vi "RMSE_Rotation.vi"(7 "Values":T3, 8 "mask":i32[][](array[numeric]), 9 "rev/s":dbl, 10 "Coord Grid":cdb[][](array[numeric]), 11 "V m/s":cdb[][][](array[numeric])) -> ()   [LabVIEW 2022 SP3]
uses:
  <vilib>/Utility/miscctls.llb/LVPointDoubleTypeDef.ctl
  <vilib>/Analysis/5stat.llb/RMS (DBL).vi
  <vilib>/Analysis/2dsp.llb/Decimate (single shot, DBL).vi
  <vilib>/Utility/file.llb/Write Delimited Spreadsheet (DBL).vi
  <vilib>/Analysis/NI_AALPro.lvlib
  <vilib>/Analysis/NI_AALBase.lvlib
panel:
  in  "Angles":i32[](array[numeric])=[0, 45]
  in  "multi angles":bool
  in  "Xtra Data Shift":T1
  out "ideal V cm/s":dbl[][](graph)
  in  "Tab Control":T2(tab)
  out "A1 Mean phase":dbl[][](graph)
  out "A1 Mean Vx":dbl[][](graph)
  out "AMean Vy":dbl[][](graph)
  out "A1 Mean V":dbl[][](graph)
  out "A2 Mean V":dbl[][](graph)
  out "A2 Mean Vy":dbl[][](graph)
  out "A2 Mean Vx":dbl[][](graph)
  out "A2 Mean phase":dbl[][](graph)
  out "Angles":i32[](array[numeric])
  out "ideal V_y cm/s 2":dbl[][](graph)
  out "ideal V_y cm/s":dbl[][](graph)
  out "ideal V_xcm/s":dbl[][](graph)
  out "RMSE V cm/s":dbl[][](graph)
  out "RMSE Phase (degrees)":dbl[][](graph)
  out "RMSE V_x cm/s":dbl[][](graph)
  out "RMSE  V_y cm/s":dbl[][](graph)
  out "Mean V cm/s":dbl[][](graph)
  out "Mean Phase":dbl[][](graph)
  out "Mean V _x cm/s":dbl[][](graph)
  out "Mean V y cm/s":dbl[][](graph)
  out "SD V cm/s":dbl[][](graph)
  out "SD Phase":dbl[][](graph)
  out "SD V_x cm/s":dbl[][](graph)
  out "SD V_y cm/s":dbl[][](graph)
  in  "Save":bool
  in  "Clockwise Rotate angle":i32
  in  "Pad Pts":i32=1
  out "Average RMSE Phase":dbl
  out "Average RMSE":dbl
  out "Max V":dbl
  in  "Scale?":bool
  in  "Operation":u16(ring) items=["Median", "Mean"]
  in  "median size":dbl=3.0
  # "9 and 5 tested"
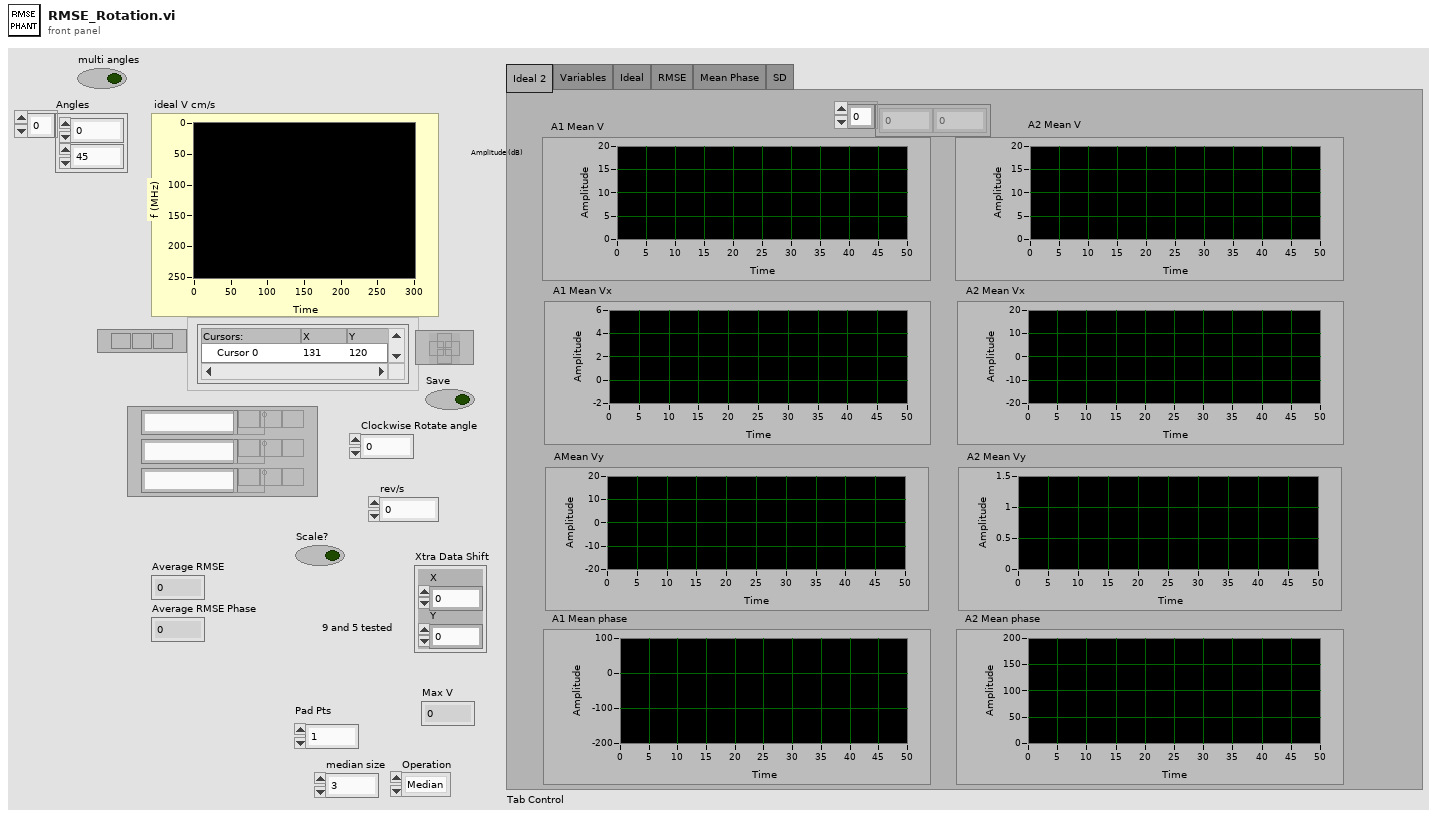
[diagram p1: front panel]
types:
  T1 = typedef "LVPointDoubleTypeDef.ctl" = cluster{"X":dbl, "Y":dbl}
  T2 = enum32{"Ideal 2", "Variables", "Ideal", "RMSE", "Mean Phase", "SD"}
  T3 = cluster{"xdim":dbl, "ydim":dbl, "zdim":dbl, "skip":dbl, "ensembleC":dbl, "ensembleVar\n":dbl, "#tx":dbl, "#Rx":dbl, "deltaX":dbl, "deltaY":dbl, "x start":dbl, "ystart":dbl}
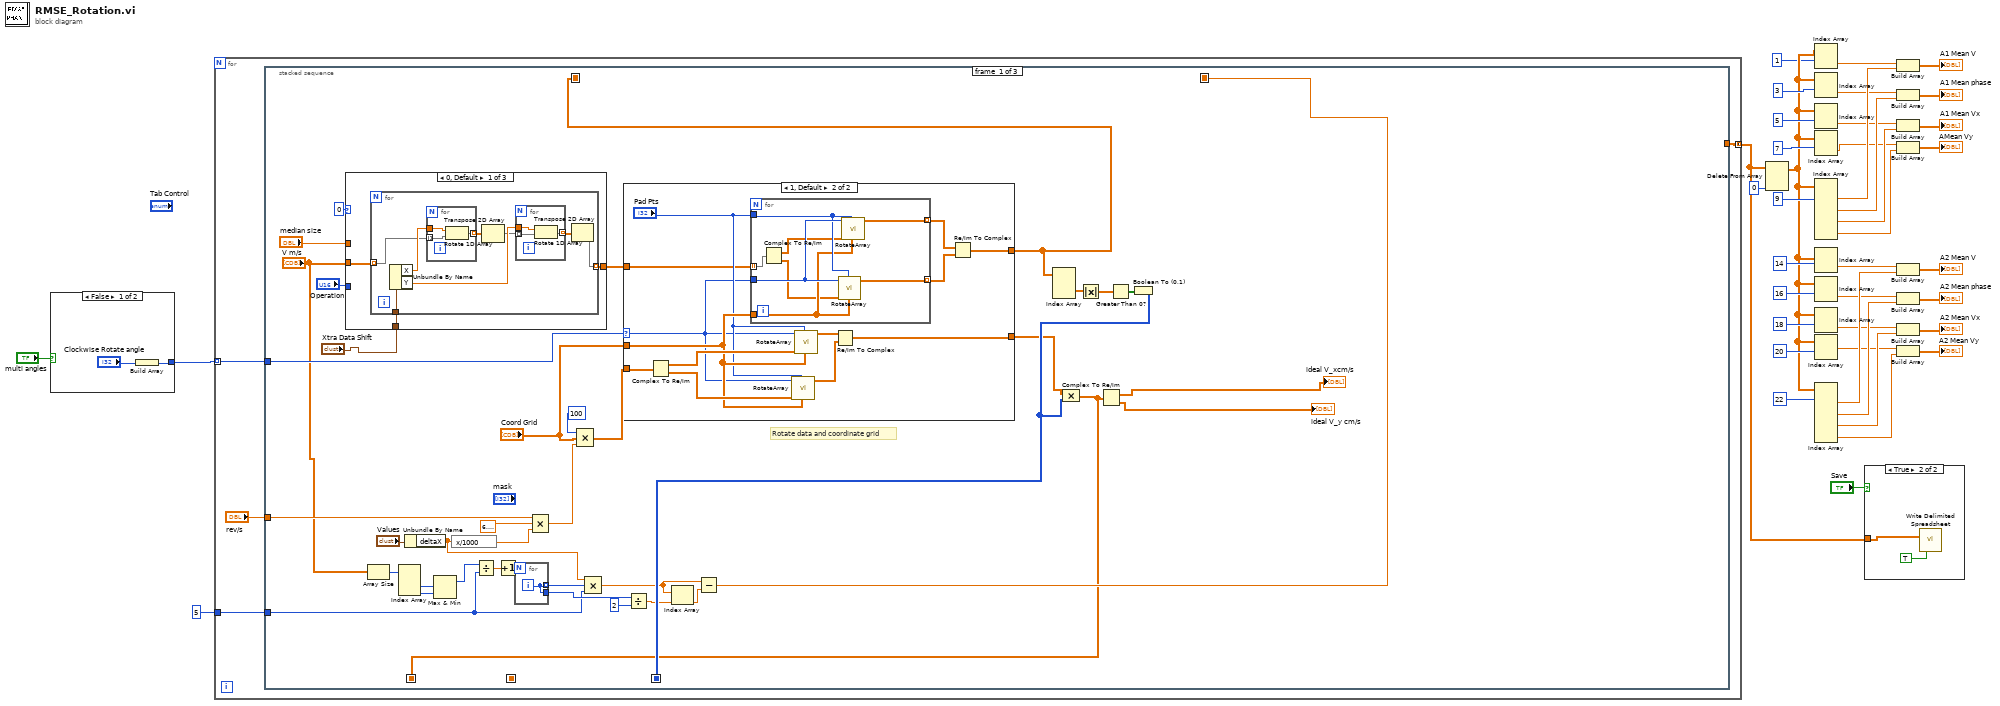
[diagram p0: block diagram]
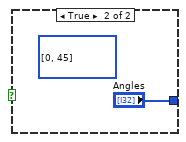
[diagram p2: hidden frame]
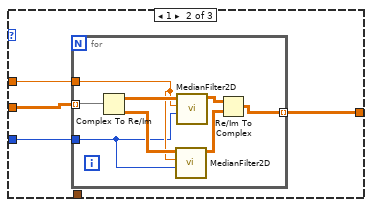
[diagram p4: hidden frame]
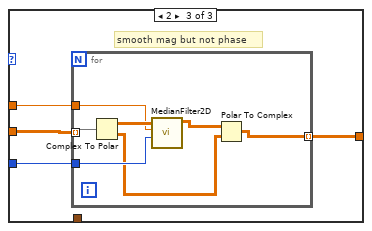
[diagram p5: hidden frame]
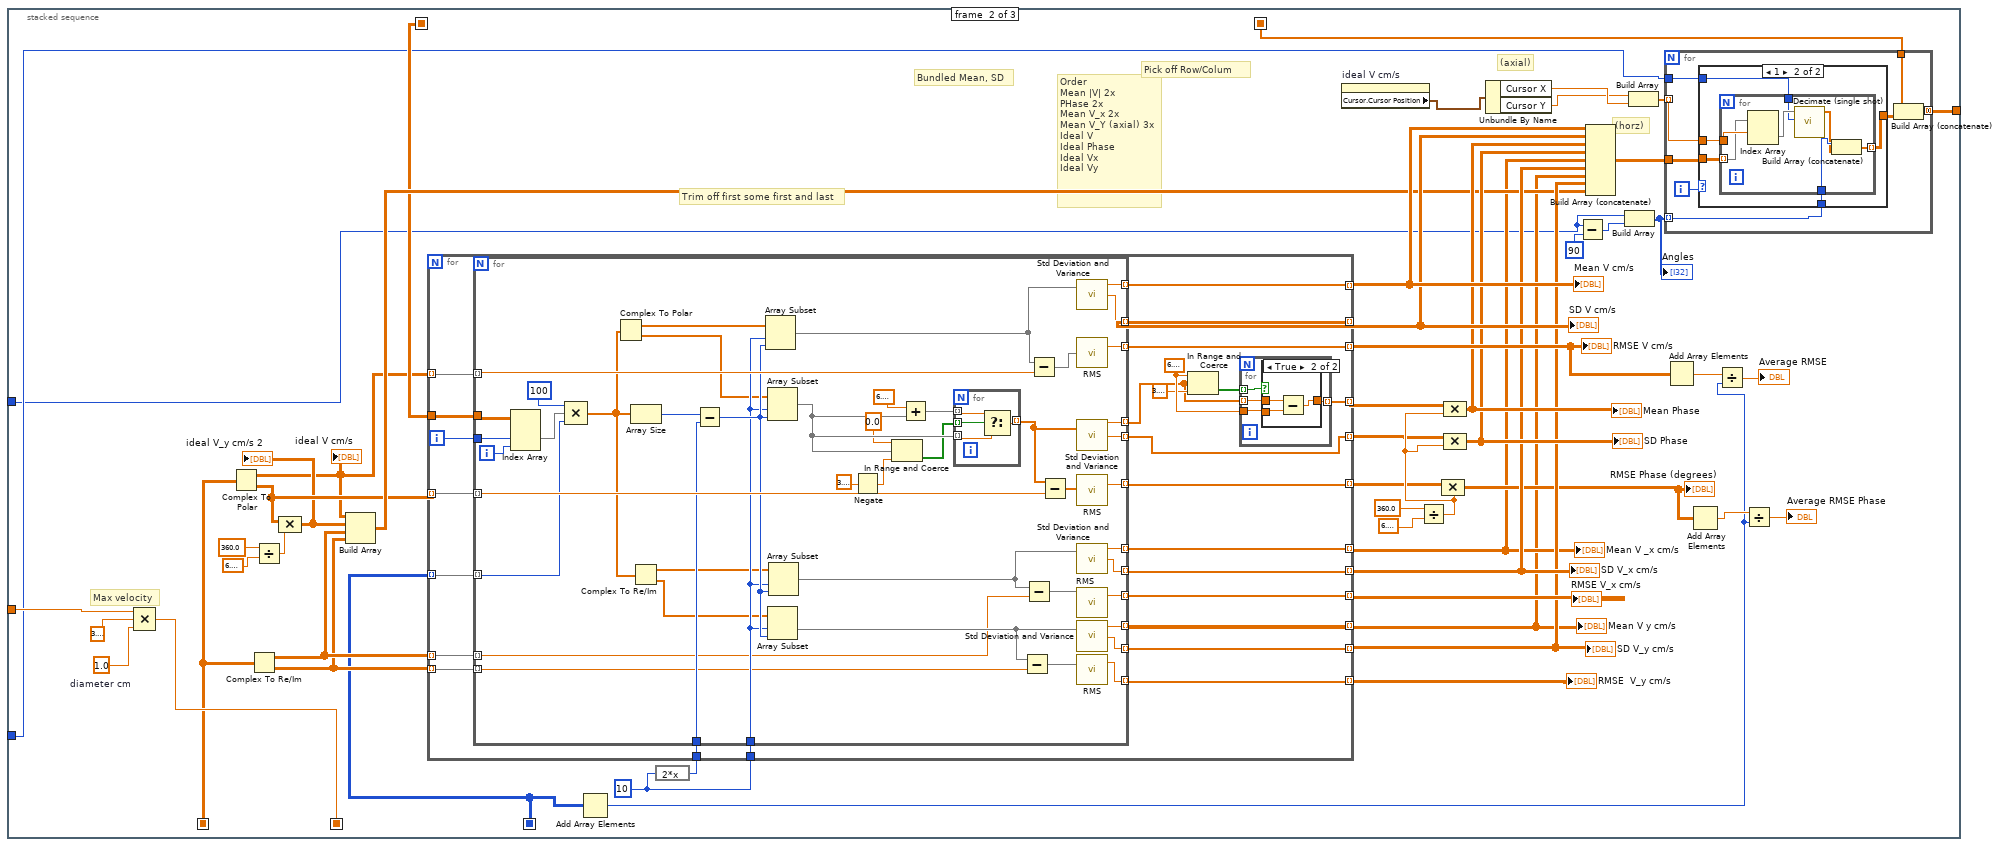
[diagram p6: hidden frame]
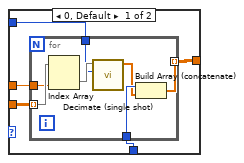
[diagram p7: hidden frame]
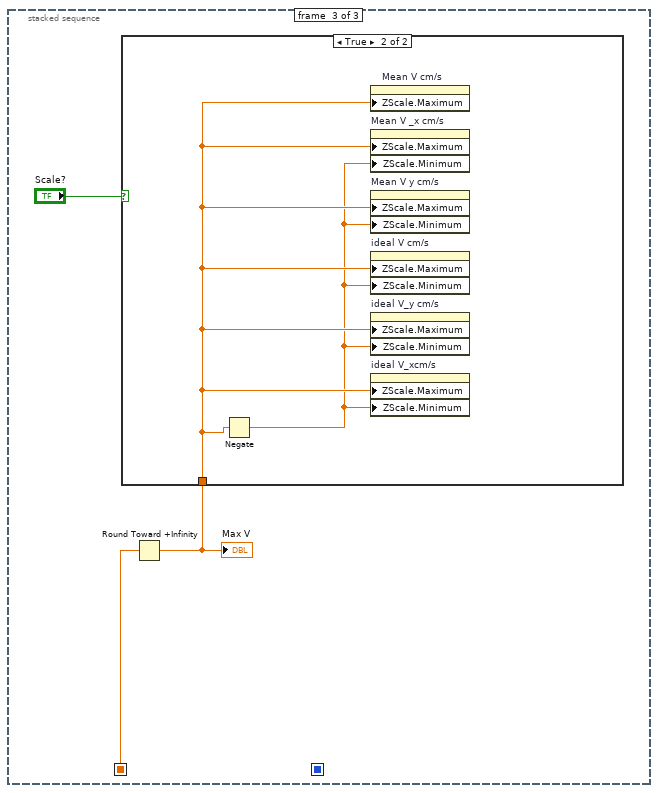
[diagram p9: hidden frame]
diagram:
  n1 = case shown="False" "multi angles" {
    tunnel: [w42 "Angles"] -> w7
    frame False {
      n2 = Build Array("Clockwise Rotate angle") -> (w42:i32[])
    }
    frame True {
      (unwired) i32[] [0, 45]
    }
  }
  n3 = for {
    tunnel: w7 -> [w47] mode=indexing
    tunnel: [w46] -> w6 mode=concatenating
    tunnel: 5 ("y") -> [w45]
    n4 = stacked-sequence {
      seq-local: [_ w170 _] -> [_ _ w321]
      seq-local: [w50 _ _] -> [_ w161 _]
      seq-local: [w73 _ _] -> [_ w168 _]
      seq-local: [w49 _ _] -> [_ w162 _]
      seq-local: [w61 _ _] -> [_ w160 _]
      tunnel: [_ w165 _] -> w46
      tunnel: "rev/s" -> [w79 w169 _]
      tunnel: w47 -> [w70 w158 _]
      tunnel: w45 -> [w53 w159 _]
      frame #0 {
        # "Rotate data and coordinate grid"
        n5 = case shown="0, Default" 0 {
          tunnel: "V m/s" -> [w114 w132 w144]
          tunnel: "median size" -> [_ w131 w143]
          tunnel: "Operation" -> [_ w130 w142]
          tunnel: [w113 w129 w141] -> w87
          tunnel: "Xtra Data Shift" -> [w112 _ _]
          frame 0, Default {
            n6 = for {
              tunnel: w114 -> [w117] mode=indexing
              tunnel: [w116] -> w113 mode=indexing
              tunnel: w112 -> [w115]
              n7 = Unbundle By Name(w115) -> ("X"=w121:dbl, "Y"=w122:dbl)
              n8 = for {
                tunnel: [w128] -> w118 mode=indexing
                tunnel: w121 -> [w127]
                tunnel: w117 -> [w126] mode=indexing
                n9 = Rotate 1D Array(1:w126, 2:w127) -> (0:w128:cdb[])
              }
              n10 = Transpose 2D Array(2D array=w118) -> (transposed array=w119:cdb[][])
              n11 = for {
                tunnel: w119 -> [w125] mode=indexing
                tunnel: [w124] -> w120 mode=indexing
                tunnel: w122 -> [w123]
                n12 = Rotate 1D Array(1:w125, 2:w123) -> (0:w124:cdb[])
              }
              n13 = Transpose 2D Array(2D array=w120) -> (transposed array=w116:cdb[][])
            }
          }
          frame 1 {
            n14 = for {
              tunnel: w132 -> [w140] mode=indexing
              tunnel: w131 -> [w134]
              tunnel: w130 -> [w133]
              tunnel: [w137] -> w129 mode=indexing
              n15 = Complex To Re/Im(x + iy=w140) -> (x=w139:dbl[][], y=w136:dbl[][])
              n16 = call "MedianFilter2D.vi"("Operation"=w133, "Pts to use"=w134, "Raw In"=w136) -> ("output array"=w135:sgl[][])  [unwired: 8 in]
              n17 = call "MedianFilter2D.vi"("Operation"=w133, "Pts to use"=w134, "Raw In"=w139) -> ("output array"=w138:sgl[][])  [unwired: 8 in]
              n18 = Re/Im To Complex(1:w135, 2:w138) -> (0:w137:csg[][])
            }
          }
          frame 2 {
            # "smooth mag but not phase"
            n19 = for {
              tunnel: w144 -> [w151] mode=indexing
              tunnel: w143 -> [w147]
              tunnel: w142 -> [w146]
              tunnel: [w148] -> w141 mode=indexing
              n20 = Complex To Polar(r * e^(i*theta)=w151) -> (r=w150:dbl[][], theta=w145:dbl[][])
              n21 = call "MedianFilter2D.vi"("Operation"=w146, "Pts to use"=w147, "Raw In"=w150) -> ("output array"=w149:sgl[][])  [unwired: 8 in]
              n22 = Polar To Complex(1:w145, 2:w149) -> (0:w148:cdb[][])
            }
          }
        }
        n23 = Array Size(array="V m/s") -> (size(s)=w59:i32[])
        n24 = Index Array(array=w59) -> (element #2=w56:i32, element #3=w55:i32)  [unwired: 3 in, 1 out]
        n25 = Unbundle By Name("Values") -> ("deltaX"=w67:dbl)
        n26 = Max & Min(x=w56, y=w55) -> (max(x,y)=w54:i32)  [unwired: 1 out]
        n27 = expression code="x/1000"(w67) -> (w80:dbl)
        n28 = Divide(x=w54, y=w53) -> (x/y=w58:dbl)
        n29 = Increment(x=w58) -> (x+1=w57:dbl)
        n30 = for {
          N: w57 -> [_]
          tunnel: [w88] -> w68 mode=indexing
          tunnel: [w88] -> w66
          i -> [w88]
        }
        n31 = Compound Arithmetic op=MULTIPLY(w79, 6.283185307179586, w80) -> (w77:dbl)
        n32 = Compound Arithmetic op=MULTIPLY(100, "Coord Grid", w77) -> (w69:cdb[][])
        n33 = Compound Arithmetic op=MULTIPLY(w67, w68, w53) -> (w63:dbl[])
        n34 = case shown="1, Default" w70 {
          selector: w70 -> [_ w93]
          tunnel: w87 -> [w90 w91]
          tunnel: [w90 w101] -> w50
          tunnel: "Coord Grid" -> [_ w95]
          tunnel: [w89 w96] -> w51
          tunnel: w69 -> [w89 w92]
          frame 0 {
          }
          frame 1, Default {
            n35 = Complex To Re/Im(x + iy=w92) -> (x=w100:dbl[][], y=w99:dbl[][])
            n36 = for {
              tunnel: [w111] -> w103 mode=indexing
              tunnel: [w110] -> w102 mode=indexing
              tunnel: w93 -> [w109]
              tunnel: w95 -> [w107]
              tunnel: "Pad Pts" -> [w108]
              tunnel: w91 -> [w104] mode=indexing
              n37 = Complex To Re/Im(x + iy=w104) -> (x=w106:dbl[][], y=w105:dbl[][])
              n38 = call "RotateArray.vi"("Vel grid Ideal"=w107, "Pad Pts"=w108, "Peak V in"=w105, "Angle"=w109) -> ("Peak V out"=w110:dbl[][])  [unwired: 6 in, 1 out]
              n39 = call "RotateArray.vi"("Vel grid Ideal"=w107, "Pad Pts"=w108, "Peak V in"=w106, "Angle"=w109) -> ("Peak V out"=w111:dbl[][])  [unwired: 6 in, 1 out]
            }
            n40 = call "RotateArray.vi"("Vel grid Ideal"=w95, "Pad Pts"="Pad Pts", "Peak V in"=w99, "Angle"=w93) -> ("Peak V out"=w97:dbl[][])  [unwired: 6 in, 1 out]
            n41 = call "RotateArray.vi"("Vel grid Ideal"=w95, "Pad Pts"="Pad Pts", "Peak V in"=w100, "Angle"=w93) -> ("Peak V out"=w98:dbl[][])  [unwired: 6 in, 1 out]
            n42 = Re/Im To Complex(1:w97, 2:w98) -> (0:w96:cdb[][])
            n43 = Re/Im To Complex(1:w102, 2:w103) -> (0:w101:cdb[][][])
          }
        }
        n44 = Divide(x=w66, y=2) -> (x/y=w64:dbl)
        n45 = Index Array(array=w63, index=w64) -> (element=w62:dbl)
        n46 = Subtract(x=w63, y=w62) -> (x-y=w61:dbl[])
        n47 = Index Array(array=w50) -> (element=w76:cdb[][])  [unwired: 3 in]
        n48 = Absolute Value(x=w76) -> (abs(x)=w75:dbl[][])
        n49 = Greater Than 0?(x=w75) -> (x > 0?=w74:bool[][])
        n50 = Boolean To (0,1)(Boolean=w74) -> (0, 1=w73:i16[][])
        n51 = Compound Arithmetic op=MULTIPLY(w51, w73) -> (w49:cdb[][])
        n52 = Complex To Re/Im(x + iy=w49) -> (x=→"ideal V_xcm/s":dbl[][], y=→"ideal V_y cm/s":dbl[][])
      }
      frame #1 {
        w171 = 1.0  # diameter cm
        w201 = 10
        # "(horz)"
        # "(axial)"
        # "Pick off Row/Colum"
        # "Order\nMean |V| 2x\nPHase 2x\nMean V_x 2x\nMean V_Y (axial) 3x\nIdeal V\nIdeal Phase\nIdeal Vx\nIdeal Vy"
        # "Bundled Mean, SD"
        # "Max velocity"
        # "Trim off first some first and last"
        n53 = Compound Arithmetic op=MULTIPLY(w169, 3.141592653589793, w171) -> (w170:dbl)
        n54 = Complex To Polar(r * e^(i*theta)=w162) -> (r=w152:dbl[][], theta=w154:dbl[][])
        "ideal V cm/s" <- w152
        n55 = Complex To Re/Im(x + iy=w162) -> (x=w177:dbl[][], y=w176:dbl[][])
        n56 = Divide(x=360.0, y=6.283185307179586) -> (x/y=w179:dbl)
        n57 = Compound Arithmetic op=MULTIPLY(w154, w179) -> (w153:dbl[][])
        "ideal V_y cm/s 2" <- w153
        n58 = Build Array(w152, w153, w177, w176) -> (w178:dbl[][][])
        n59 = Add Array Elements(numeric array=w168) -> (sum=w195:i16)
        n60 = expression code="2*x"(w201) -> (w202:i32)
        n61 = for {
          tunnel: [w245] -> w192 mode=indexing
          tunnel: [w260] -> w188 mode=indexing
          tunnel: w152 -> [w259] mode=indexing
          tunnel: w154 -> [w258] mode=indexing
          tunnel: w202 -> [w257]
          tunnel: w201 -> [w256]
          tunnel: [w244] -> w194 mode=indexing
          tunnel: [w255] -> w193 mode=indexing
          tunnel: [w239] -> w173 mode=indexing
          tunnel: [w238] -> w191 mode=indexing
          tunnel: [w254] -> w186 mode=indexing
          tunnel: [w253] -> w175 mode=indexing
          tunnel: [w252] -> w184 mode=indexing
          tunnel: [w251] -> w174 mode=indexing
          tunnel: [w250] -> w185 mode=indexing
          tunnel: [w249] -> w187 mode=indexing
          tunnel: w168 -> [w248] mode=indexing
          tunnel: w177 -> [w247] mode=indexing
          tunnel: w176 -> [w246] mode=indexing
          tunnel: w161 -> [w243]
          i -> [w261]
          w241 = 6.283185307179586
          n62 = for {
            tunnel: w243 -> [w315]
            tunnel: w261 -> [w314]
            tunnel: [w311] -> w245 mode=indexing
            tunnel: [w310] -> w260 mode=indexing
            tunnel: w259 -> [w309] mode=indexing
            tunnel: w258 -> [w308] mode=indexing
            tunnel: w257 -> [w306]
            tunnel: w256 -> [w298]
            tunnel: [w303] -> w244 mode=indexing
            tunnel: [w300] -> w255 mode=indexing
            tunnel: [w302] -> w237 mode=indexing
            tunnel: [w301] -> w238 mode=indexing
            tunnel: [w291] -> w254 mode=indexing
            tunnel: [w290] -> w253 mode=indexing
            tunnel: [w283] -> w252 mode=indexing
            tunnel: [w286] -> w251 mode=indexing
            tunnel: [w285] -> w250 mode=indexing
            tunnel: [w284] -> w249 mode=indexing
            tunnel: w248 -> [w280] mode=indexing
            tunnel: w247 -> [w282] mode=indexing
            tunnel: w246 -> [w281] mode=indexing
            i -> [w313]
            n63 = Index Array(array=w315, index (dim 1)=w314, index (dim 2)=w313) -> (element=w289:cdb[])  [unwired: 1 in]
            n64 = Compound Arithmetic op=MULTIPLY(100, w289, w280) -> (w287:cdb[])
            n65 = Complex To Polar(r * e^(i*theta)=w287) -> (r=w305:dbl[], theta=w271:dbl[])
            n66 = Array Size(array=w287) -> (size(s)=w307:i32)
            n67 = Complex To Re/Im(x + iy=w287) -> (x=w297:dbl[], y=w296:dbl[])
            n68 = Subtract(x=w307, y=w306) -> (x-y=w299:i32)
            n69 = Array Subset(array=w305, index=w298, length=w299) -> (w304:dbl[])
            n70 = Array Subset(array=w271, index=w298, length=w299) -> (w275:dbl[])
            n71 = Array Subset(array=w296, index=w298, length=w299) -> (w293:dbl[])
            n72 = Array Subset(array=w297, index=w298, length=w299) -> (w292:dbl[])
            n73 = Negate(x=3.141592653589793) -> (-x=w276:dbl)
            n74 = In Range and Coerce(upper limit=0.0, x=w275, lower limit=w276) -> (In Range?=w274:bool[])  [unwired: 1 out]
            n75 = Add(x=6.283185307179586, y=w275) -> (x+y=w273:dbl[])
            n76 = for {
              tunnel: w274 -> [w319] mode=indexing
              tunnel: w275 -> [w317] mode=indexing
              tunnel: w273 -> [w318] mode=indexing
              tunnel: [w316] -> w272 mode=indexing
              n77 = Select(t=w318, s=w319, f=w317) -> (s? t:f=w316:dbl)
            }
            n78 = Subtract(x=w293, y=w281) -> (x-y=w294:dbl[])
            n79 = Subtract(x=w292, y=w282) -> (x-y=w295:dbl[])
            n80 = Subtract(x=w304, y=w309) -> (x-y=w279:dbl[])
            n81 = Subtract(x=w272, y=w308) -> (x-y=w312:dbl[])
            n82 = call <vilib>:"Std Deviation and Variance.vi"("X"=w304) -> ("mean"=w303:dbl, "standard deviation"=w300:dbl)  [unwired: 1 in, 1 out]
            n83 = call-poly <vilib>:"RMS.vi"("X"=w279) -> ("rms value"=w311:dbl)  [unwired: 1 out]
            n84 = call <vilib>:"Std Deviation and Variance.vi"("X"=w272) -> ("mean"=w302:dbl, "standard deviation"=w301:dbl)  [unwired: 1 in, 1 out]
            n85 = call-poly <vilib>:"RMS.vi"("X"=w312) -> ("rms value"=w310:dbl)  [unwired: 1 out]
            n86 = call <vilib>:"Std Deviation and Variance.vi"("X"=w292) -> ("mean"=w290:dbl, "standard deviation"=w284:dbl)  [unwired: 1 in, 1 out]
            n87 = call-poly <vilib>:"RMS.vi"("X"=w295) -> ("rms value"=w291:dbl)  [unwired: 1 out]
            n88 = call <vilib>:"Std Deviation and Variance.vi"("X"=w293) -> ("mean"=w286:dbl, "standard deviation"=w285:dbl)  [unwired: 1 in, 1 out]
            n89 = call-poly <vilib>:"RMS.vi"("X"=w294) -> ("rms value"=w283:dbl)  [unwired: 1 out]
          }
          n90 = In Range and Coerce(upper limit=w241, x=w237, lower limit=3.141592653589793) -> (In Range?=w242:bool[])  [unwired: 1 out]
          n91 = for {
            tunnel: w242 -> [w265] mode=indexing
            tunnel: [w264] -> w239 mode=indexing
            tunnel: w241 -> [w263]
            tunnel: w237 -> [w262] mode=indexing
            n92 = case shown="True" w265 {
              tunnel: [w266 w269] -> w264
              tunnel: w263 -> [_ w268]
              tunnel: w262 -> [w266 w267]
              frame False {
              }
              frame True {
                n93 = Subtract(x=w267, y=w268) -> (x-y=w269:dbl)
              }
            }
          }
        }
        "RMSE V cm/s" <- w192
        "Mean V cm/s" <- w194
        "SD V cm/s" <- w193
        "RMSE V_x cm/s" <- w186
        "SD V_x cm/s" <- w187
        "Mean V _x cm/s" <- w175
        "RMSE  V_y cm/s" <- w184
        "Mean V y cm/s" <- w174
        "SD V_y cm/s" <- w185
        n94 = property on="ideal V cm/s" class="IntGraph (strict)"() -> ("Cursor.Cursor Position"=w155:T1)  [unwired: 2 in, 2 out]
        n95 = Divide(x=360.0, y=6.283185307179586) -> (x/y=w200:dbl)
        n96 = Compound Arithmetic op=MULTIPLY(w188, w200) -> (w183:dbl[][])
        "RMSE Phase (degrees)" <- w183
        n97 = Compound Arithmetic op=MULTIPLY(w173, w200) -> (w190:dbl[][])
        "Mean Phase" <- w190
        n98 = Compound Arithmetic op=MULTIPLY(w191, w200) -> (w189:dbl[][])
        "SD Phase" <- w189
        n99 = Unbundle By Name(w155) -> ("Cursor X"=w164:dbl, "Cursor Y"=w163:dbl)
        n100 = Subtract(x=w158, y=90) -> (x-y=w156:i32)
        n101 = Build Array (concatenate)(w194, w193, w190, w189, w175, w187, w174, w185, w178) -> (w182:dbl[][][])
        n102 = Build Array(w158, w156) -> (w166:i32[])
        "Angles" <- w166
        n103 = Build Array(w163, w164) -> (w167:dbl[])
        n104 = for {
          tunnel: w182 -> [w212]
          tunnel: [w206] -> w165 mode=concatenating
          tunnel: w167 -> [w211] mode=indexing
          tunnel: w166 -> [w209] mode=indexing
          tunnel: w160 -> [w207]
          tunnel: w159 -> [w205]
          i -> [w210]
          n105 = case shown="1" w210 {
            tunnel: w212 -> [w216 w228]
            tunnel: w211 -> [w217 w229]
            tunnel: [w215 w227] -> w208
            tunnel: w209 -> [w214 w226]
            tunnel: w205 -> [w213 w225]
            frame 0, Default {
              n106 = for {
                tunnel: w217 -> [w223]
                tunnel: w216 -> [w224] mode=indexing
                tunnel: [w221] -> w215 mode=indexing
                tunnel: w214 -> [w222]
                tunnel: w213 -> [w218]
                n107 = Index Array(array=w224, index (col)=w223) -> (element=w220:dbl[])  [unwired: 1 in]
                n108 = call-poly <vilib>:"Decimate (single shot).vi"("decimating factor"=w218, "X"=w220) -> ("Decimated Array"=w219:dbl[])  [unwired: 8 in, 1 out]
                n109 = Build Array (concatenate)(w222, w219) -> (w221:dbl[])
              }
            }
            frame 1 {
              n110 = for {
                tunnel: w229 -> [w236]
                tunnel: w228 -> [w235] mode=indexing
                tunnel: [w233] -> w227 mode=indexing
                tunnel: w226 -> [w234]
                tunnel: w225 -> [w230]
                n111 = Index Array(array=w235, index (row)=w236) -> (element=w232:dbl[])  [unwired: 1 in]
                n112 = call-poly <vilib>:"Decimate (single shot).vi"("decimating factor"=w230, "X"=w232) -> ("Decimated Array"=w231:dbl[])  [unwired: 8 in, 1 out]
                n113 = Build Array (concatenate)(w234, w231) -> (w233:dbl[])
              }
            }
          }
          n114 = Build Array (concatenate)(w207, w208) -> (w206:dbl[][])
        }
        n115 = Add Array Elements(numeric array=w192) -> (sum=w199:dbl)
        n116 = Add Array Elements(numeric array=w183) -> (sum=w198:dbl)
        n117 = Divide(x=w199, y=w195) -> (x/y=→"Average RMSE":dbl)
        n118 = Divide(x=w198, y=w195) -> (x/y=→"Average RMSE Phase":dbl)
      }
      frame #2 {
        n119 = Round Toward +Infinity(x=w321) -> (ceil(x): smallest int >= x=w320:dbl)
        "Max V" <- w320
        n120 = case shown="True" "Scale?" {
          tunnel: w320 -> [_ w324]
          frame False {
          }
          frame True {
            n121 = Negate(x=w324) -> (-x=w323:dbl)
            n122 = property on="Mean V cm/s" class="IntGraph (strict)"("ZScale.Maximum"=w324) -> ()  [unwired: 2 in, 2 out]
            n123 = property on="Mean V _x cm/s" class="IntGraph (strict)"("ZScale.Maximum"=w324, "ZScale.Minimum"=w323) -> ()  [unwired: 2 in, 2 out]
            n124 = property on="Mean V y cm/s" class="IntGraph (strict)"("ZScale.Maximum"=w324, "ZScale.Minimum"=w323) -> ()  [unwired: 2 in, 2 out]
            n125 = property on="ideal V cm/s" class="IntGraph (strict)"("ZScale.Maximum"=w324, "ZScale.Minimum"=w323) -> ()  [unwired: 2 in, 2 out]
            n126 = property on="ideal V_y cm/s" class="IntGraph (strict)"("ZScale.Maximum"=w324, "ZScale.Minimum"=w323) -> ()  [unwired: 2 in, 2 out]
            n127 = property on="ideal V_xcm/s" class="IntGraph (strict)"("ZScale.Maximum"=w324, "ZScale.Minimum"=w323) -> ()  [unwired: 2 in, 2 out]
          }
        }
      }
    }
  }
  n128 = Delete From Array(array=w6, index (col)=0 ("disabled index (col)")) -> (array with subset deleted=w4:dbl[][])  [unwired: 2 in, 1 out]
  n129 = Index Array(array=w4, index (row)=1) -> (element=w35:dbl[])  [unwired: 1 in]
  n130 = Index Array(array=w4, index (row)=3 ("disabled index (col)")) -> (element=w33:dbl[])  [unwired: 1 in]
  n131 = Index Array(array=w4, index (row)=5 ("disabled index (col)")) -> (element=w26:dbl[])  [unwired: 1 in]
  n132 = Index Array(array=w4, index (row)=7 ("disabled index (col)")) -> (element=w25:dbl[])  [unwired: 1 in]
  n133 = Index Array(array=w4, index (row) #1=9 ("disabled index (col)")) -> (element #1=w34:dbl[], element #2=w32:dbl[], element #3=w31:dbl[], element #4=w30:dbl[])  [unwired: 7 in]
  n134 = Index Array(array=w4, index (row)=14 ("disabled index (col)")) -> (element=w20:dbl[])  [unwired: 1 in]
  n135 = Index Array(array=w4, index (row)=16 ("disabled index (col)")) -> (element=w18:dbl[])  [unwired: 1 in]
  n136 = Index Array(array=w4, index (row)=18 ("disabled index (col)")) -> (element=w14:dbl[])  [unwired: 1 in]
  n137 = Index Array(array=w4, index (row)=20 ("disabled index (col)")) -> (element=w13:dbl[])  [unwired: 1 in]
  n138 = Index Array(array=w4, index (row) #1=22 ("disabled index (col)")) -> (element #1=w19:dbl[], element #2=w17:dbl[], element #3=w16:dbl[], element #4=w15:dbl[])  [unwired: 7 in]
  n139 = case shown="True" "Save" {
    tunnel: w6 -> [_ w326]
    frame False {
    }
    frame True {
      n140 = call-poly <vilib>:"Write Delimited Spreadsheet.vi"("2D data"=w326, "transpose? (no:F)"=TRUE) -> ()  [unwired: 12 in, 2 out]
    }
  }
  n141 = Build Array(w35, w34) -> (→"A1 Mean V":dbl[][])
  n142 = Build Array(w33, w32) -> (→"A1 Mean phase":dbl[][])
  n143 = Build Array(w26, w31) -> (→"A1 Mean Vx":dbl[][])
  n144 = Build Array(w25, w30) -> (→"AMean Vy":dbl[][])
  n145 = Build Array(w20, w19) -> (→"A2 Mean V":dbl[][])
  n146 = Build Array(w18, w17) -> (→"A2 Mean phase":dbl[][])
  n147 = Build Array(w14, w16) -> (→"A2 Mean Vx":dbl[][])
  n148 = Build Array(w13, w15) -> (→"A2 Mean Vy":dbl[][])
